vi "Pack Control Message.vi"(10 "Controller Message Type":T1, 11 "Controller":T2) -> (3 "Controller Message out":refnum<class "Controller Message.lvclass">)   [LabVIEW 2015, in "RDS Controller Actor.lvlib"]
uses:
  RDS Controller Actor.lvlib
  Libraries/RDS Child Messages/Controller Message/Controller Message.lvclass
  Controller.ctl
  Libraries/RDS Child Messages/Controller Message/Controller Message Type.ctl
  Libraries/RDS Framework/RDS Message ID.ctl
  Libraries/RDS Framework/RDS Message Class/RDS Message.lvclass/RDS Message.ctl
  Libraries/RDS Child Messages/Controller Message/Controller Message.lvclass/Controller Message.ctl
  Libraries/RDS Child Messages/RDS Child Messages.lvlib
  Libraries/RDS Framework/RDS Message Class/RDS Message.lvclass
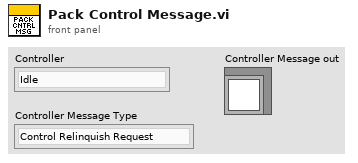
[diagram p1: front panel]
types:
  T1 = typedef "RDS Child Messages.lvlib/Controller Message.lvclass/Controller Message Type.ctl" = enum16{"Control Relinquish Request", "Control Relinquish Command", "Control Request", "Control Granted"}
  T2 = typedef "RDS Controller Actor.lvlib/Controller.ctl" = enum16{"Idle", "Local Remote Control", "Shore Remote Control", "Mission Control"}
  T3 = typedef "RDS Child Messages.lvlib/RDS Message ID.ctl" = enum16{"RDS Hello World", "String Message", "AIP_Status", "AIP_Command", "GPS_Data", "MCB_Command", "MCB_Status", "Compass_Data", "Depth_Data", "Battery_Data", "Contoller_State", "Set_Mag_Dev", "BTB_Shutdown", "State_Sample_Request", "State_Sample", "PID_Gains_Set", "Helm_Limiter_Set", "Helm_Heading_Command", "Helm_Steering_Command", "Helm_Status", "Controller_Message", "AIP_Set_Min_Depth", "Mission_Controller_State", "Mission_Upload", "Mission_Set_Op_and_Run", "Mission_Settings_Set"}
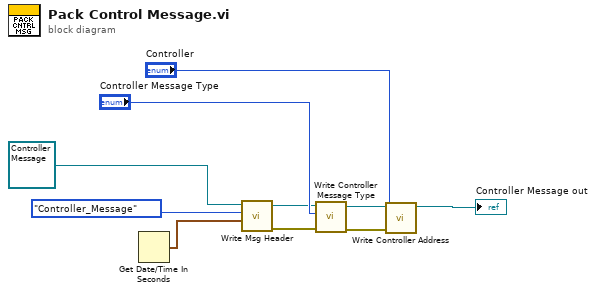
[diagram p0: block diagram]
diagram:
  n1 = Get Date/Time In Seconds() -> (seconds since 1Jan1904=w2:timestamp)
  n2 = call "Write Msg Header.vi"("Time Stamp"=w2, "Msg ID"=RDS_Message_ID."Controller_Message" ("RDS Message"), "RDS Message in"=refnum<class "Controller Message.lvclass"> refnum ("RDS Child Messages.lvlib:Controller Message.lvclass")) -> ("error out"=w8:errorcluster, "RDS Message out"=w4:refnum<class "Controller Message.lvclass">)  [unwired: 7 in]
  n3 = call "Write Controller Message Type.vi"("error in (no error)"=w8, "Controller Message Type"="Controller Message Type", "Controller Message in"=w4) -> ("error out"=w9:errorcluster, "Controller Message out"=w6:refnum<class "Controller Message.lvclass">)  [unwired: 7 in]
  n4 = call "Write Controller Address.vi"("error in (no error)"=w9, "Controller"="Controller", "Controller Message in"=w6) -> ("Controller Message out"=→"Controller Message out":refnum<class "Controller Message.lvclass">)  [unwired: 7 in, 1 out]
